vi "LMS_RecvStream.vi"(6 "meta":T2, 8 "error in (no error)":errorcluster, 9 "timeout_ms":u64, 10 "stream":T1, 11 "sample_count":u64) -> (0 "error out":errorcluster, 1 "samples":dbl[](array[numeric]))   [LabVIEW 2013, in "LMS_LV_Drv.lvlib"]
uses:
  LMS_LV_Drv.lvlib
  Stream_ctl.ctl
  LimeSuite.dll
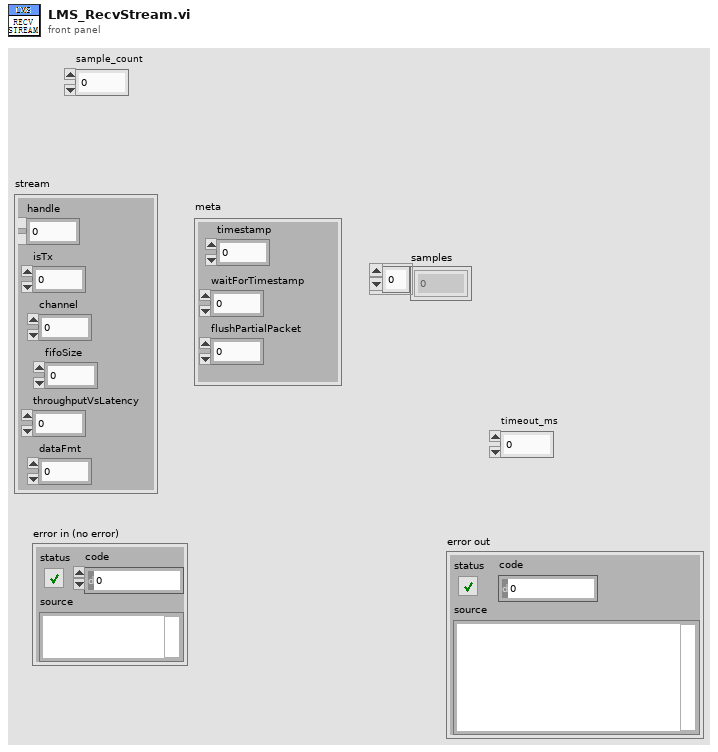
[diagram p1: front panel]
types:
  T1 = typedef "Stream_ctl.ctl" = cluster{"handle":u64, "isTx":u8, "channel":u32, "fifoSize":u32, "throughputVsLatency":dbl, "dataFmt":u32}
  T2 = cluster{"timestamp":u64, "waitForTimestamp":u8, "flushPartialPacket":u8}
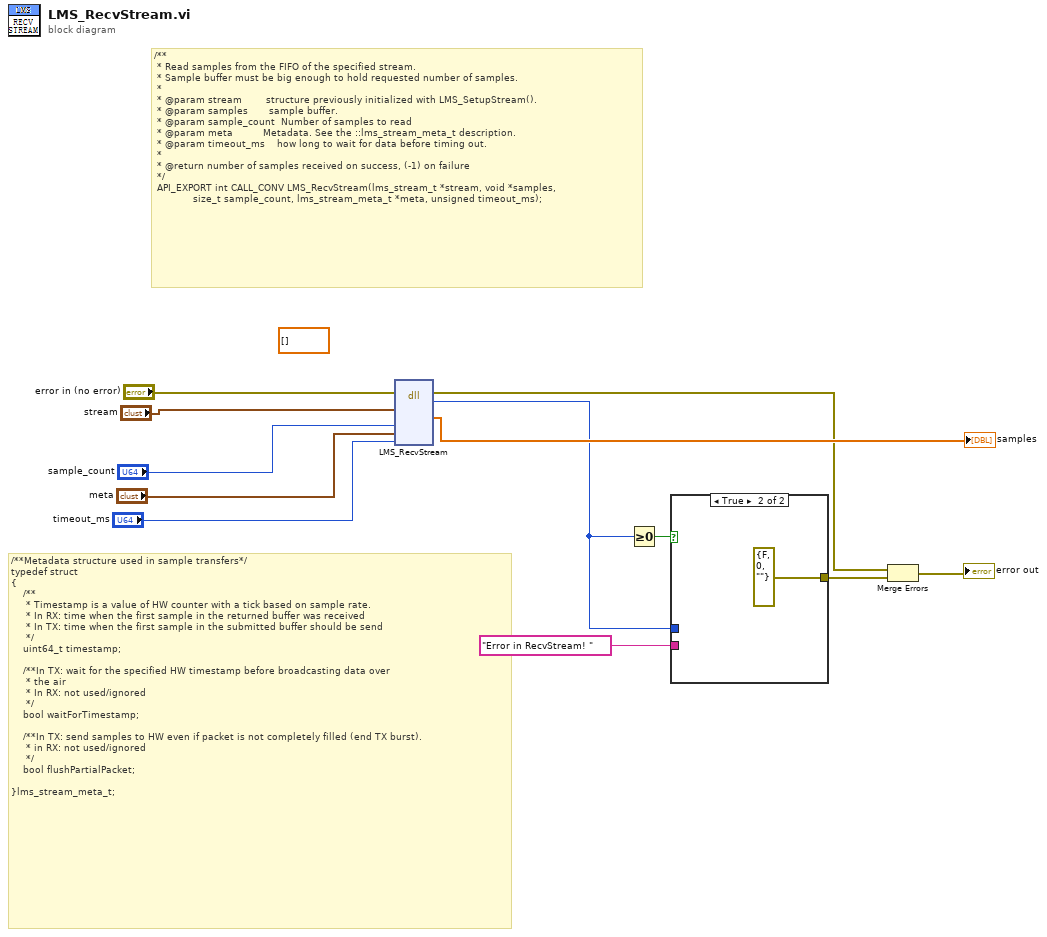
[diagram p0: block diagram]
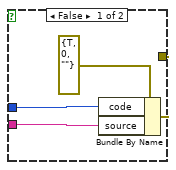
[diagram p2: hidden frame]
diagram:
  (unwired) sgl[] [] ("samples")
  # "/**Metadata structure used in sample transfers*/\ntypedef struct\n{\n    /**\n     * Timestamp is a value of HW counter with a tick based on sample rate.\n     * In RX: time when the first sample in the returned buffer was received\n     * In TX: time when the first sample in the submitted buffer should be send\n     */\n    uint64_t timestamp;\n\n    /**In TX: wait for the specified HW timestamp before broadcasting data over\n     * the air\n     * In RX: not used/ignored\n     */\n    bool waitForTimestamp;\n\n    /**In TX: send samples to HW even if packet is not completely filled (end TX burst).\n     * in RX: not used/ignored\n     */\n    bool flushPartialPacket;\n\n}lms_stream_meta_t;"
  # "/**\n * Read samples from the FIFO of the specified stream.\n * Sample buffer must be big enough to hold requested number of samples.\n *\n * @param stream        structure previously initialized with LMS_SetupStream().\n * @param samples       sample buffer.\n * @param sample_count  Number of samples to read\n * @param meta          Metadata. See the ::lms_stream_meta_t description.\n * @param timeout_ms    how long to wait for data before timing out.\n *\n * @return number of samples received on success, (-1) on failure\n */\n API_EXPORT int CALL_CONV LMS_RecvStream(lms_stream_t *stream, void *samples,\n             size_t sample_count, lms_stream_meta_t *meta, unsigned timeout_ms);"
  n1 = dll-call lib="PTH1mabs CUsersOTADesktop书籍出版程序8.第八章LimeSDR_LabVIEW_Driver-master\nLimeSuite.dll" fn="LMS_RecvStream"(error in="error in (no error)", "steam"="stream", "sample_count"="sample_count", "meta"="meta", "timeout_ms"="timeout_ms") -> (error out=w2:errorcluster, "return type"=w3:i32, "samples"=→"samples":sgl[])  [unwired: 7 in, 1 out]
  n2 = Greater Or Equal To 0?(x=w3) -> (x >= 0?=w6:bool)
  n3 = case shown="True" w6 {
    tunnel: [w15 errorcluster {"status"=FALSE, "code"=0, "source"=""} ("error in")] -> w4
    tunnel: w3 -> [w14 _]
    tunnel: "Error in RecvStream! " ("source") -> [w13 _]
    frame False {
      n4 = Bundle By Name(cluster=errorcluster {"status"=TRUE, "code"=0, "source"=""} ("error in"), "code"=w14, "source"=w13) -> (w15:errorcluster)
    }
    frame True {
    }
  }
  n5 = Merge Errors(w2, w4) -> (→"error out":errorcluster)
